vi "Get Accelerometer.vi"() -> (0 "Accelerations":T1)   [LabVIEW 2014]
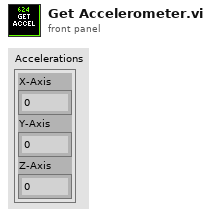
[diagram p1: front panel]
types:
  T1 = cluster{"X-Axis":dbl, "Y-Axis":dbl, "Z-Axis":dbl}
  T2 = typedef "WPI_AccelerometerDevRef.ctl" = cluster{"DevStatus":errorcluster, "Controller":T3, "Scaling":T4, "Analog Channels":T5, "I2C Bus":T7, "SPI Bus":T8, "Accel Range":T9, "ADXL345 Axes":T10, "Handle":i32, "Device Address":u8, "Accel Type":enum16{"Analog", "ADXL345 I2C", "ADXL345 SPI", "Internal"}}
  T3 = typedef "FPGA_TypedefAnalogModule.ctl" = enum16{"Controller 1"}
  T4 = typedef "WPI_AccelerometerScaling.ctl" = cluster{"Gain (VoltsPerG)":dbl, "Center Voltage":dbl}
  T5 = typedef "WPI_AccelerometerAnalogChannels.ctl" = cluster{"X-Axis":T6, "Y-Axis":T6, "Z-Axis":T6}
  T6 = typedef "FPGA_AIChannel.ctl" = enum8{"AI 0", "AI 1", "AI 2", "AI 3", "AI MXP 0", "AI MXP 1", "AI MXP 2", "AI MXP 3", "Invalid"}
  T7 = typedef "i2c_bus.ctl" = enum16{"I2C On-Board", "I2C MXP", "Invalid"}
  T8 = typedef "spi_bus.ctl" = enum16{"SPI On-Board, CS0", "SPI On-Board, CS1", "SPI On-Board, CS2", "SPI On-Board, CS3", "SPI MXP", "Invalid"}
  T9 = typedef "ADXL345 Range.ctl" = u8
  T10 = typedef "WPI_AccelerometerADXL345 Axes.ctl" = cluster{"X-Axis":bool, "Y-Axis":bool, "Z-Axis":bool}
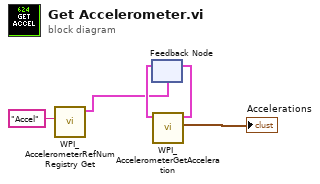
[diagram p0: block diagram]
diagram:
  n1 = call <vilib>:"WPI_AccelerometerRefNum Registry Get.vi"("refnum name"="Accel") -> ("AccelerometerDevRef"=w2:T2)  [unwired: 9 in, 1 out]
  n2 = feedback #1(w2) -> (w3:T2)
  n3 = call <vilib>:"WPI_AccelerometerGetAcceleration.vi"("AccelerometerDevRef"=w3) -> ("Accelerations"=→"Accelerations":T1, "AccelerometerDevRef"=w4:T2)  [unwired: 8 in, 1 out]
  n4 = feedback-in #1(w4) -> ()
